vi "SPI_WriteBytes.vi"(5 "Device":i32, 6 "Bytes":u8[](array[numeric]) format="%.0x", 7 "Bus":i32=1, 8 "error in":errorcluster) -> (0 "error out":errorcluster)   [LabVIEW 2014, in "GPIO.lvlib"]
doc: "Write bytes to the specified device"
uses:
  GPIO.lvlib
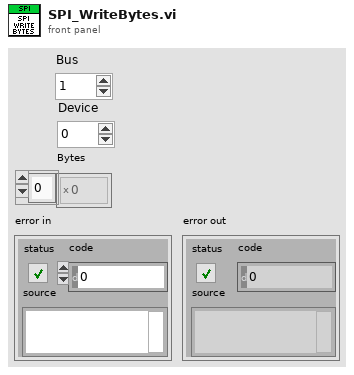
[diagram p1: front panel]
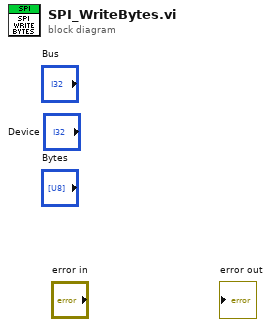
[diagram p0: block diagram]
diagram:
